vi "Variancia_online.vi"(8 "error in (no error)":errorcluster, 10 "M":dbl, 11 "u":dbl) -> (0 "error out":errorcluster, 1 "std":dbl, 2 "var":dbl, 3 "y":dbl)   [LabVIEW 2019]
panel:
  in  "Tab Control":enum32{"Page 1", "Page 2"}(tab)
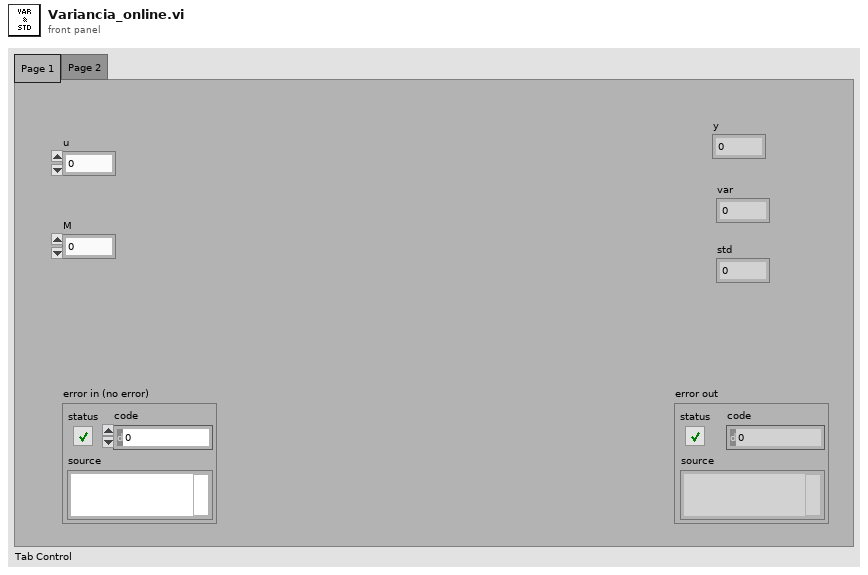
[diagram p1: front panel]
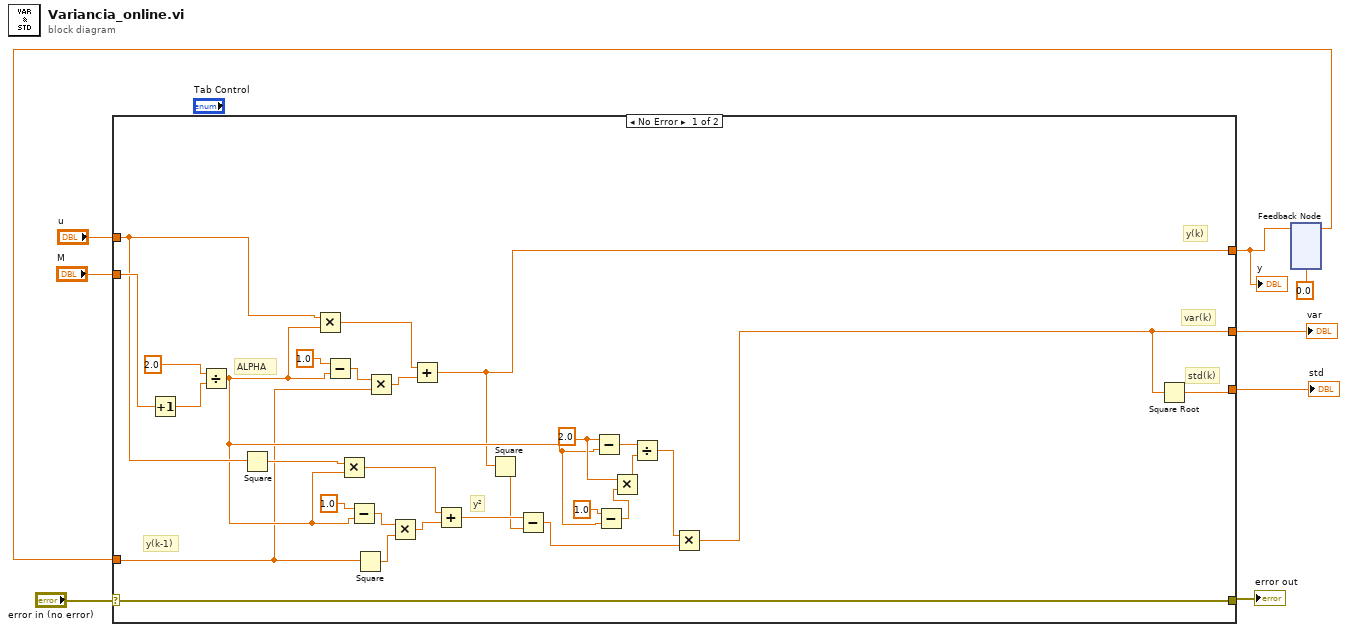
[diagram p0: block diagram]
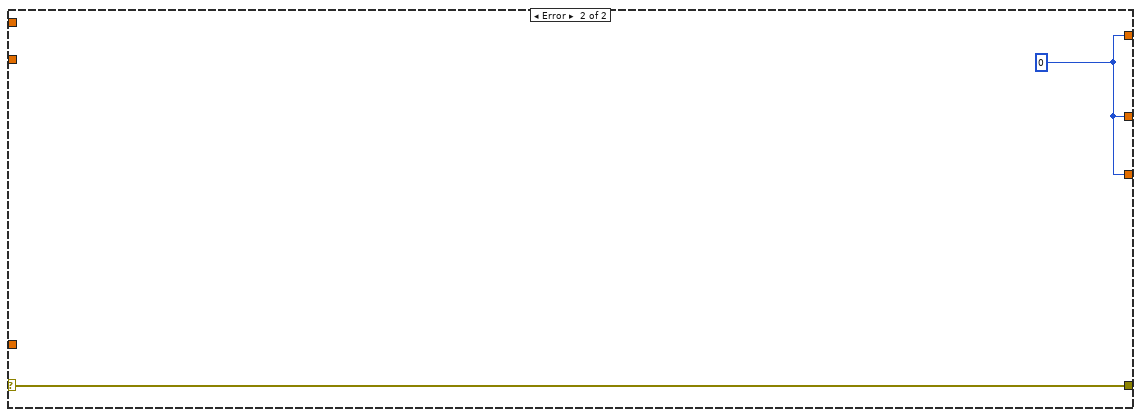
[diagram p2: hidden frame]
diagram:
  n1 = feedback #1(0.0) -> (w3:dbl)
  n2 = case shown="No Error" "error in (no error)" {
    selector: "error in (no error)" -> [w38 w40]
    tunnel: "M" -> [w35 _]
    tunnel: "u" -> [w25 _]
    tunnel: [w38 w40] -> w6
    tunnel: [w17 w39] -> w1
    tunnel: [w11 w39] -> w5
    tunnel: [w12 w39] -> w4
    tunnel: w3 -> [w10 _]
    frame No Error {
      w22 = 2.0
      # "std(k)"
      # "var(k)"
      # "y(k)"
      # "y(k-1)"
      # "y²"
      # "ALPHA"
      n3 = Increment(x=w35) -> (x+1=w36:dbl)
      n4 = Divide(x=2.0, y=w36) -> (x/y=w20:dbl)
      n5 = Square(x=w25) -> (x^2=w24:dbl)
      n6 = Multiply(x=w25, y=w20) -> (x*y=w31:dbl)
      n7 = Subtract(x=1.0, y=w20) -> (x-y=w34:dbl)
      n8 = Multiply(x=w24, y=w20) -> (x*y=w30:dbl)
      n9 = Subtract(x=1.0, y=w20) -> (x-y=w27:dbl)
      n10 = Square(x=w10) -> (x^2=w26:dbl)
      n11 = Multiply(x=w34, y=w10) -> (x*y=w33:dbl)
      n12 = Multiply(x=w27, y=w26) -> (x*y=w28:dbl)
      n13 = Add(x=w31, y=w33) -> (x+y=w17:dbl)
      n14 = Add(x=w30, y=w28) -> (x+y=w16:dbl)
      n15 = Square(x=w17) -> (x^2=w15:dbl)
      n16 = Subtract(x=w16, y=w15) -> (x-y=w14:dbl)
      n17 = Subtract(x=w22, y=w20) -> (x-y=w23:dbl)
      n18 = Subtract(x=1.0, y=w20) -> (x-y=w19:dbl)
      n19 = Multiply(x=w22, y=w19) -> (x*y=w18:dbl)
      n20 = Divide(x=w23, y=w18) -> (x/y=w13:dbl)
      n21 = Multiply(x=w13, y=w14) -> (x*y=w11:dbl)
      n22 = Square Root(x=w11) -> (sqrt(x)=w12:dbl)
    }
    frame Error {
      w39 = 0
    }
  }
  "y" <- w1
  "error out" <- w6
  "std" <- w4
  "var" <- w5
  n23 = feedback-in #1(w1) -> ()
